vi "GC_GaN.vi"() -> ()   [LabVIEW 2011]
uses:
  DynaGlbs.vi
  ScrnGlbs.vi
  SysGlbs.vi
  TimeGlbs.vi
  SpecGlbs.vi
  RcpGlbs.vi
  RobotGlbs.vi
panel:
  out "PP Rout":string="Pump Purge Rout"
  out "shutter_indicator":string
  in  "32":bool
  in  "91":bool
  in  "92":bool
  in  "97":bool
  in  "101":bool
  in  "108":bool
  in  "123":bool
  out "val102 2":bool
  in  "Fout25":dbl min=0.0 max=5000.0 format="%.1f"
  in  "Fout29":dbl min=0.0 max=5000.0 format="%.1f"
  in  "Fout30":dbl min=0.0 max=5000.0 format="%.1f"
  in  "Fout26":dbl min=0.0 max=5000.0 format="%.1f"
  in  "Fout52":dbl min=0.0 max=5000.0 format="%.1f"
  in  "Fout53":dbl min=0.0 max=5000.0 format="%.1f"
  in  "Fout54":dbl min=0.0 max=5000.0 format="%.1f"
  in  "Fout38":dbl min=0.0 max=5000.0 format="%.1f"
  in  "Fout41":dbl min=0.0 max=5000.0 format="%.1f"
  in  "Fout49":dbl min=0.0 max=5000.0 format="%.1f"
  in  "Fout50":dbl min=0.0 max=5000.0 format="%.1f"
  in  "Fout51":dbl min=0.0 max=5000.0 format="%.1f"
  in  "Fout73":dbl min=0.0 max=5000.0 format="%.1f"
  in  "Fout87":dbl min=0.0 max=5000.0 format="%.1f"
  in  "Fout84":dbl min=0.0 max=5000.0 format="%.1f"
  in  "Fout83":dbl min=0.0 max=5000.0 format="%.1f"
  in  "Fout88":dbl min=0.0 max=5000.0 format="%.1f"
  in  "Fout74":dbl min=0.0 max=5000.0 format="%.1f"
  in  "Fout75":dbl min=0.0 max=5000.0 format="%.1f"
  in  "Fout76":dbl min=0.0 max=5000.0 format="%.1f"
  in  "Fout85":dbl min=0.0 max=5000.0 format="%.1f"
  in  "Fout55":dbl min=0.0 max=5000.0 format="%.1f"
  out "Fin84":dbl format="%.1f"
  out "Fin88":dbl format="%.1f"
  out "Fin83":dbl format="%.1f"
  out "Fin87":dbl format="%.1f"
  out "Fin86":dbl format="%.1f"
  out "Fin85":dbl format="%.1f"
  out "Fin92":dbl format="%.1f"
  out "Fin93":dbl format="%.1f"
  out "Fin94":dbl format="%.1f"
  out "Fin60":dbl format="%.3e"
  out "Fin61":dbl format="%.3e"
  out "Fin65":dbl format="%.1f"
  out "Fin73":dbl format="%.1f"
  out "Fin66":dbl format="%.1f"
  out "Fin67":dbl format="%.1f"
  out "Fin68":dbl format="%.1f"
  out "Fin69":dbl format="%.1f"
  out "Fin70":dbl format="%.1f"
  out "Fin74":dbl format="%.1f"
  out "Fin75":dbl format="%.1f"
  out "Fin76":dbl format="%.1f"
  out "Fin27":dbl format="%.1f"
  out "Fin29 2":dbl format="%.1f"
  out "Fin30 2":dbl format="%.1f"
  out "Fin38 2":dbl format="%.1f"
  out "Fin42 2":dbl format="%.1f"
  out "Fin52":dbl format="%.1f"
  out "Fin53":dbl format="%.1f"
  out "Fin54":dbl format="%.1f"
  out "Fin43":dbl format="%.1f"
  out "Fin41 2":dbl format="%.1f"
  out "Fin25 2":dbl format="%.1f"
  out "Fin26 2":dbl format="%.1f"
  out "Fin40":dbl format="%.1f"
  out "Fin49":dbl format="%.1f"
  out "Fin50":dbl format="%.1f"
  out "Fin51":dbl format="%.1f"
  out "Fin28":dbl format="%.1f"
  out "Fin55":dbl format="%.1f"
  in  "104":bool
  in  "ChgPW":bool
  in  "111":bool
  in  "110":bool
  in  "109":bool
  in  "112":bool
  in  "54":bool
  in  "Scrn Btns":T1
  out "bub8":string="TMAl #2"
  out "bub7":string="TMGa"
  out "bub6":string="TEGa"
  out "bub5":string="TMIn #2"
  out "bub4":string="TMIn #1"
  out "bub3":string="TMAl #1"
  out "bub2":string="Cp2Mg"
  out "bub1":string="DEZn"
  out "gas2":string="SiH4"
  in  "panel location and size":T2={"left"=0, "top"=78, "right"=887, "bottom"=700}
  in  "37":bool
  in  "38":bool
  in  "34":bool
  in  "36":bool
  in  "33":bool
  in  "35":bool
  in  "43":bool
  out "Vac lock":string="locked"
  out "LL lock":string="locked"
  out "GV lock":string="locked"
  in  "50":bool
  in  "49":bool
  out "LL Door":bool
  in  "44":bool
  in  "46":bool
  in  "40":bool
  in  "56":bool
  in  "42":bool
  in  "93":bool
  in  "39":bool
  in  "41":bool
  in  "47":bool
  in  "26":bool
  in  "53":bool
  in  "45":bool
  in  "55":bool
  in  "GV Down":bool=TRUE
  in  "GV Up":bool
  in  "30":bool
  in  "31":bool
  in  "94":bool
  in  "51":bool
  in  "103":bool
  in  "48":bool
  in  "28":bool
  in  "val102":bool
  in  "52":bool
  # "102"
  # "INNER"
  # "MIDDLE"
  # "OUTER"
  # "VOLTAGE"
  # "CURRENT"
  # "POWER"
  # "VIEW PORT\n   SHIELD"
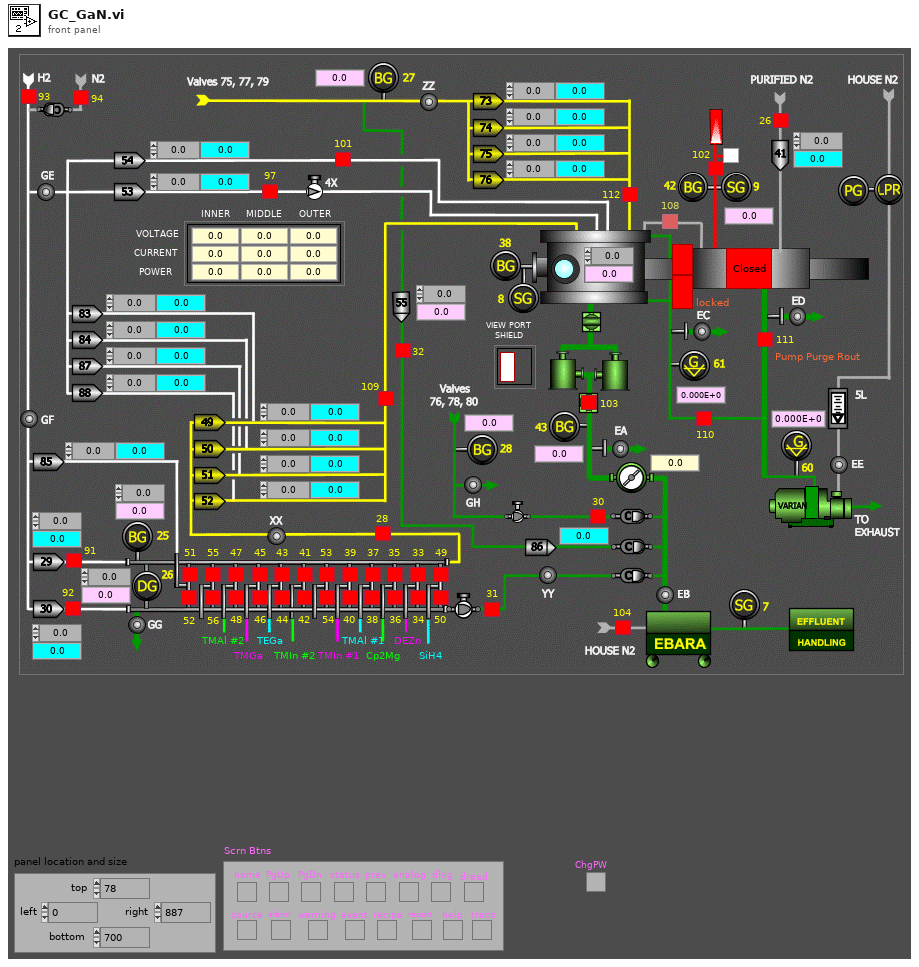
[diagram p1: front panel]
types:
  T1 = cluster{"home":bool, "PgUp":bool, "PgDn":bool, "status":bool, "prev":bool, "analog":bool, "dlog":bool, "dread":bool, "source":bool, "alarm":bool, "warning":bool, "event":bool, "recipe":bool, "report":bool, "help":bool, "trans":bool}
  T2 = cluster{"left":i16, "top":i16, "right":i16, "bottom":i16}
  T3 = enum16{"Load", "Read", "Open", "Close", "Invisible"}
  T4 = cluster{"Press":u8[], "PD_cell":cluster{"H2_cell":u8, "H2_line":u8, "horn":u8, "light":u8, "temp":u8, "PD_cell?":bool, "Temp Set":u16, "N2_in":u8, "N2_line":u8}, "RampDn":u8[], "GV/LL":cluster{"LL Door":u8, "GV Up":u8, "GV Low":u8, "GV _LIn":u8, "Fork":u8, "GV_UIn":u8, "GC Press":u8, "LL Press":u8, "MDA_LL":u8[], "Motor":u8, "EQ Valve":u8, "LL Active":u8}, "GC_Pump":cluster{"LL_Vac":u8, "GC_Vac":u8, "Bypass":u8, "Rough":u8, "Isolat":u8, "LL_MDA":u8[], "Vac_Press":u8, "TGV":u8}, "N2 Purge":cluster{"N2_LL":u8, "MFC":u8}, "RampRate":dbl[], "GC_Vac":cluster{"D_Vac-":u8[], "D_Vac+":u8[], "A_Vac":u8[], "D_Open+":u8[], "D_Open-":u8[], "A_Open":u8[]}, "Toxic":u8[], "Indicators":u8[], "LL Routine":cluster{"D Open":u8[], "D Close":u8[], "Timeout(ms)":u32}, "Temperature":u8[], "EBARA Pump":cluster{"EBARA_Din":cluster{"Main Status":u8, "Booster Status":u8, "Indicator":u8, "N2 Isolat":u8}, "EBARA_N2":u8[]}}
  T5 = cluster{"LL Door":u8, "GV Up":u8, "GV Low":u8, "GV _LIn":u8, "Fork":u8, "GV_UIn":u8, "GC Press":u8, "LL Press":u8, "MDA_LL":u8[], "Motor":u8, "EQ Valve":u8, "LL Active":u8}
  T6 = cluster{"[0]":dbl, "[1]":dbl, "[2]":dbl, "[3]":dbl, "[4]":dbl, "[5]":dbl}
  T7 = cluster{"[0]":dbl, "[1]":dbl, "[2]":dbl, "[3]":dbl, "[4]":dbl, "[5]":dbl, "[6]":dbl}
  T8 = cluster{"[0]":dbl, "[1]":dbl, "[2]":dbl, "[3]":dbl, "[4]":dbl, "[5]":dbl, "[6]":dbl, "[7]":dbl, "[8]":dbl, "[9]":dbl, "[10]":dbl}
  T9 = cluster{"[0]":dbl, "[1]":dbl, "[2]":dbl, "[3]":dbl}
  T10 = enum16{"Init", "Check", "TGA Status", "TGA Scrn", "Read"}
  T11 = cluster{"[0]":bool, "[1]":bool, "[2]":bool, "[3]":bool, "[4]":bool, "[5]":bool, "[6]":bool, "[7]":bool, "[8]":bool, "[9]":bool, "[10]":bool, "[11]":bool, "[12]":bool, "[13]":bool, "[14]":bool, "[15]":bool, "[16]":bool, "[17]":bool, "[18]":bool, "[19]":bool, "[20]":bool, "[21]":bool, "[22]":bool, "[23]":bool, "[24]":bool, "[25]":bool, "[26]":bool, "[27]":bool, "[28]":bool, "[29]":bool, "[30]":bool, "[31]":bool, "[32]":bool, "[33]":bool, "[34]":bool, "[35]":bool}
  T12 = cluster{"[0]":bool, "[1]":bool, "[2]":bool, "[3]":bool}
  T13 = cluster{"[0]":bool, "[1]":bool, "[2]":bool, "[3]":bool, "[4]":bool}
  T14 = cluster{"[0]":bool, "[1]":bool, "[2]":bool, "[3]":bool, "[4]":bool, "[5]":bool}
  T15 = cluster{"[0]":bool, "[1]":bool, "[2]":bool, "[3]":bool, "[4]":bool, "[5]":bool, "[6]":bool}
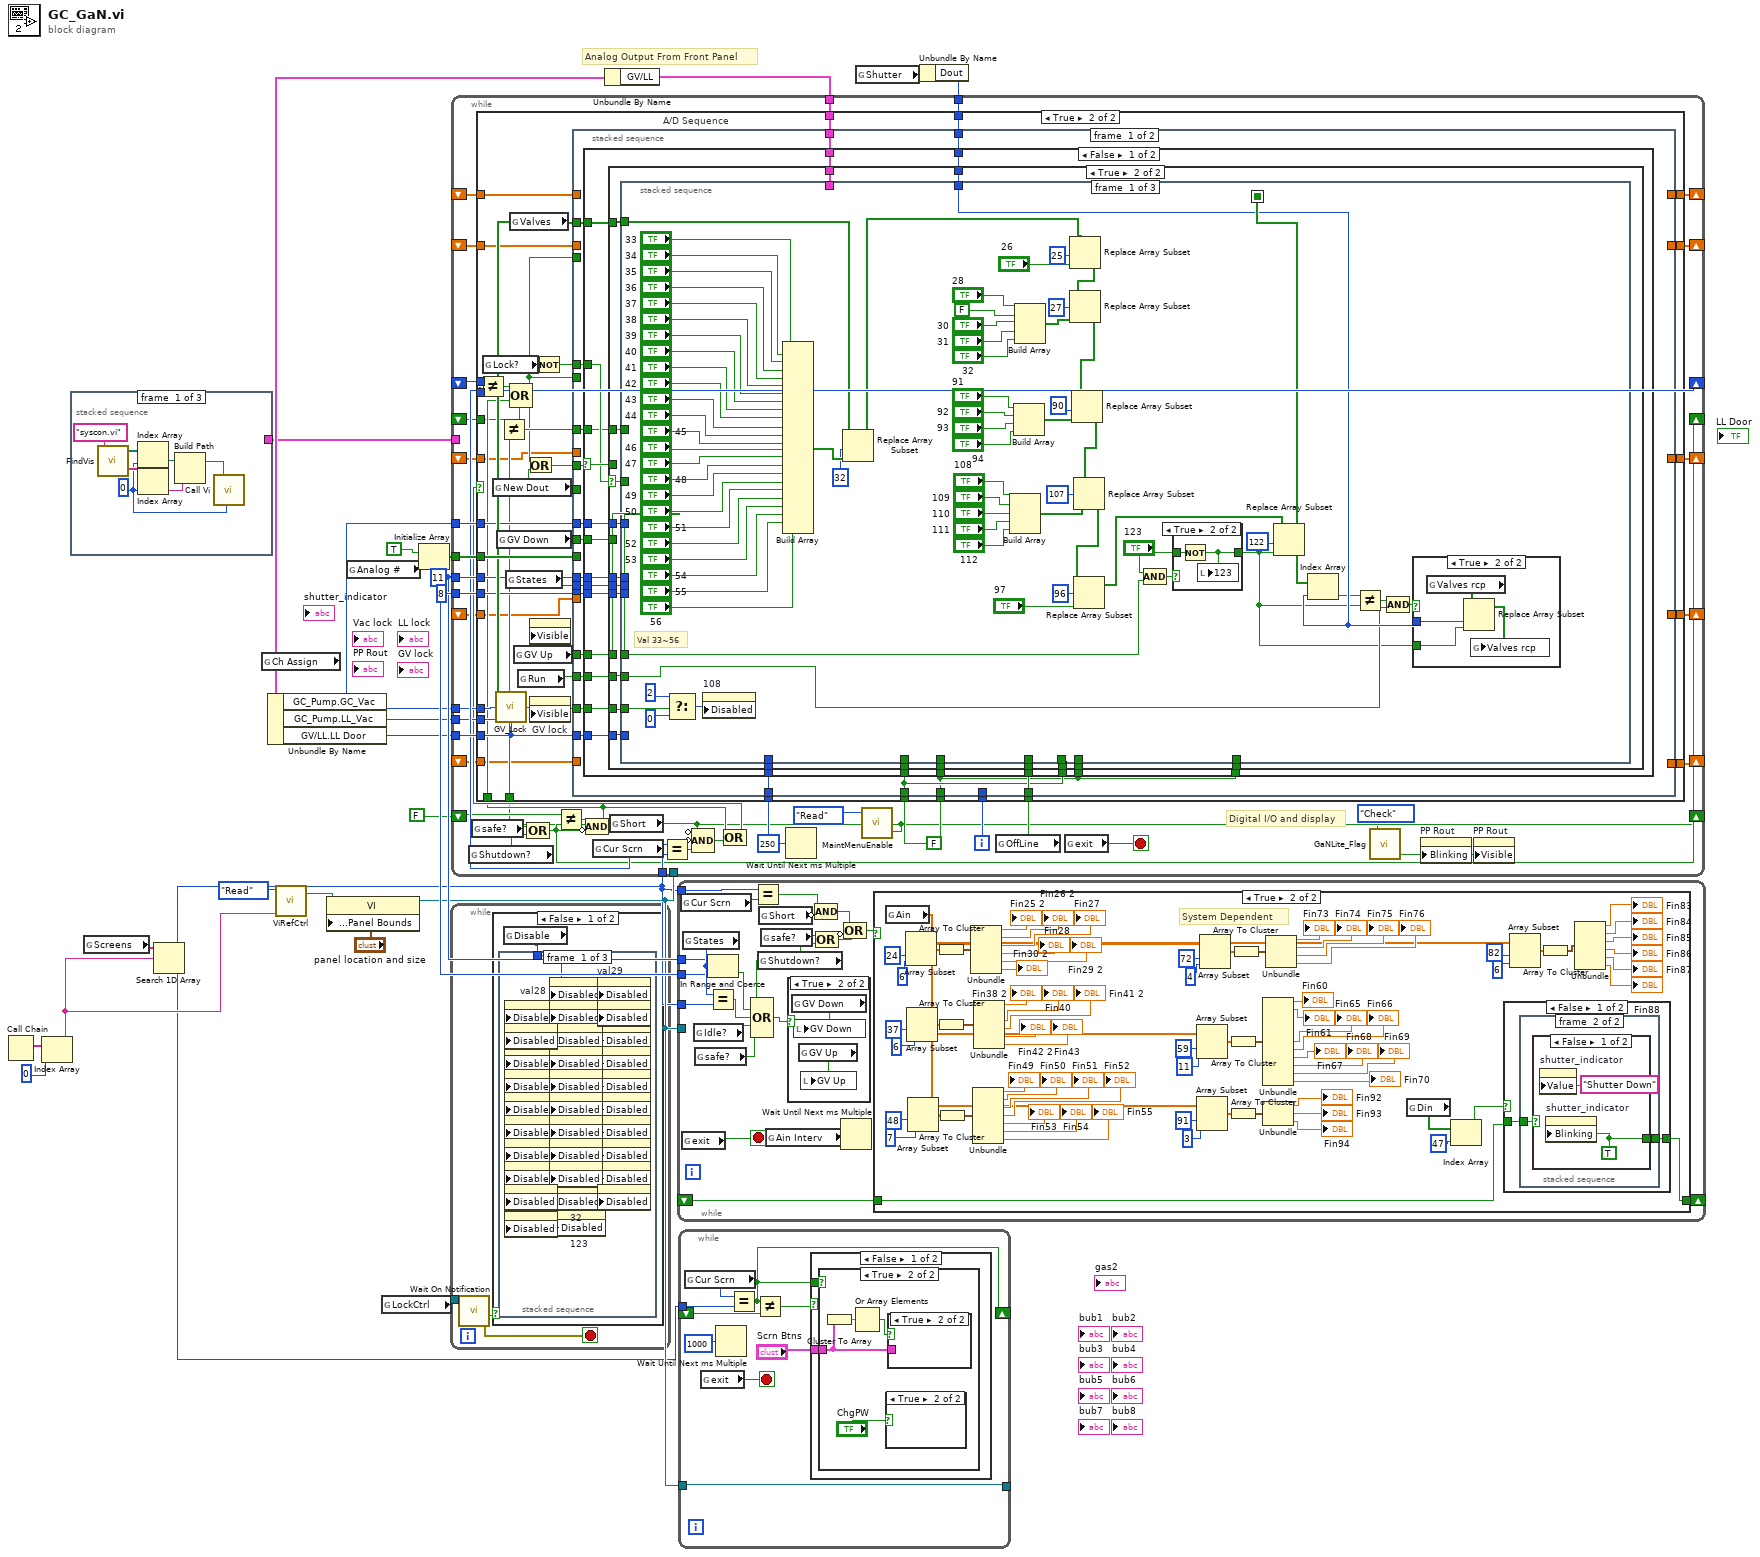
[diagram p0: block diagram]
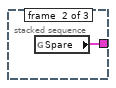
[diagram p2: hidden frame]
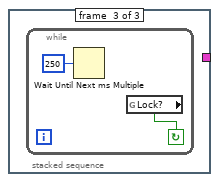
[diagram p3: hidden frame]
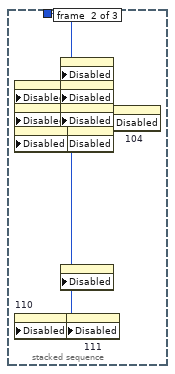
[diagram p4: hidden frame]
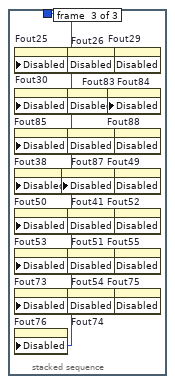
[diagram p5: hidden frame]
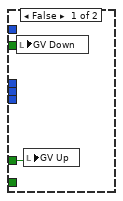
[diagram p12: hidden frame]
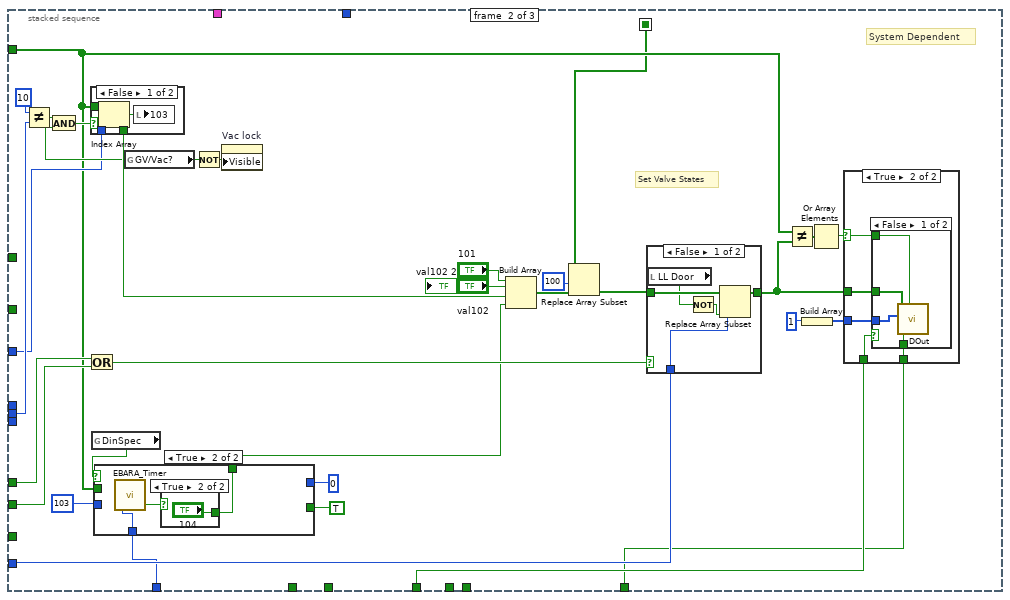
[diagram p15: hidden frame]
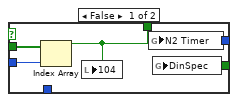
[diagram p16: hidden frame]
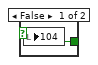
[diagram p17: hidden frame]
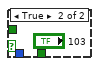
[diagram p18: hidden frame]
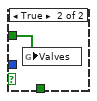
[diagram p20: hidden frame]
diagram:
  w20 = 11
  w21 = 8
  # "Analog Output From Front Panel"
  n1 = Call Chain() -> (call chain=w6:string[])
  n2 = Index Array(array=w6, index=0) -> (element=w4:string)
  n3 = stacked-sequence {
    tunnel: [_ w32 _] -> w10
    frame #0 {
      w25 = 0
      n4 = call "FindVis.vi"("Caller"="syscon.vi") -> ("Subllbs"=w30:path[], "SubVis"=w29:string[])
      n5 = Index Array(array=w30, index=w25) -> (element=w28:path)
      n6 = Index Array(array=w29, index=w25) -> (element=w27:string)
      n7 = Build Path(base path=w28, name or relative path=w27) -> (appended path=w26:path)
      n8 = call "Call Vi.vi"("call mode (open,call,close:1)"=w25, "VI path"=w26) -> ()  [unwired: 8 in, 2 out]
    }
    frame #1 {
      n9 = global read "SpecGlbs.vi" "Spare"() -> (w32:cluster{"SpareD":bool[], "SpareA":bool[]})
    }
    frame #2 {
      n10 = while {
        stop <- w34 continue-if-true
        n11 = Wait Until Next ms Multiple(millisecond multiple=u32 250) -> ()  [unwired: 1 out]
        n12 = global read "ScrnGlbs.vi" "Lock?"() -> (w34:bool)
      }
    }
  }
  n13 = global read "ScrnGlbs.vi" "Screens"() -> (w7:string[])
  n14 = Search 1D Array(1D array=w7, element=w4) -> (index of element=w3:i32)  [unwired: 1 in]
  n15 = global read "SysGlbs.vi" "Ch Assign"() -> (w13:T4)
  n16 = Unbundle By Name(w13) -> ("GC_Pump.GC_Vac"=w18:u8, "GC_Pump.LL_Vac"=w17:u8, "GV/LL.LL Door"=w16:u8)
  n17 = call "ViRefCtrl.vi"("Action"=T3."Read", "Vi Name"=w4) -> ("Vi Ref"=w14:refnum<vi>)  [unwired: 3 in, 1 out]
  n18 = property class="VI"(reference=w14, "Front Panel Window:Panel Bounds"="panel location and size") -> (reference out=w12:refnum<vi>)  [unwired: 1 in, 1 out]
  n19 = global read "SysGlbs.vi" "Analog #"() -> (w22:u32)
  n20 = global read "ScrnGlbs.vi" "LockCtrl"() -> (w11:refnum<k1>)
  n21 = Initialize Array(TRUE, w22) -> (w23:bool[])
  n22 = while {
    tunnel: w11 -> [w37]
    stop <- w35 stop-if-true
    n23 = call <vilib>:"Wait On Notification.vi"("notifier"=w37) -> ("error out"=w35:errorcluster, "timed out"=w36:bool)  [unwired: 3 in, 2 out]
    n24 = case shown="False" w36 {
      frame False {
        n25 = global read "ScrnGlbs.vi" "Disable"() -> (w38:u8)
        n26 = stacked-sequence {
          tunnel: w38 -> [w39 w40 w41]
          frame #0 {
            n27 = property on="val30" class="Bool (strict)"("Disabled"=w39) -> ()  [unwired: 2 in, 2 out]
            n28 = property on="34" class="Bool (strict)"("Disabled"=w39) -> ()  [unwired: 2 in, 2 out]
            n29 = property on="val36" class="Bool (strict)"("Disabled"=w39) -> ()  [unwired: 2 in, 2 out]
            n30 = property on="val39" class="Bool (strict)"("Disabled"=w39) -> ()  [unwired: 2 in, 2 out]
            n31 = property on="val42" class="Bool (strict)"("Disabled"=w39) -> ()  [unwired: 2 in, 2 out]
            n32 = property on="val45" class="Bool (strict)"("Disabled"=w39) -> ()  [unwired: 2 in, 2 out]
            n33 = property on="val48" class="Bool (strict)"("Disabled"=w39) -> ()  [unwired: 2 in, 2 out]
            n34 = property on="val51" class="Bool (strict)"("Disabled"=w39) -> ()  [unwired: 2 in, 2 out]
            n35 = property on="54" class="Bool (strict)"("Disabled"=w39) -> ()  [unwired: 2 in, 2 out]
            n36 = property on="112" class="Bool (strict)"("Disabled"=w39) -> ()  [unwired: 2 in, 2 out]
            n37 = property on="val28" class="Bool (strict)"("Disabled"=w39) -> ()  [unwired: 2 in, 2 out]
            n38 = property on="val31" class="Bool (strict)"("Disabled"=w39) -> ()  [unwired: 2 in, 2 out]
            n39 = property on="val37" class="Bool (strict)"("Disabled"=w39) -> ()  [unwired: 2 in, 2 out]
            n40 = property on="val40" class="Bool (strict)"("Disabled"=w39) -> ()  [unwired: 2 in, 2 out]
            n41 = property on="val43" class="Bool (strict)"("Disabled"=w39) -> ()  [unwired: 2 in, 2 out]
            n42 = property on="val46" class="Bool (strict)"("Disabled"=w39) -> ()  [unwired: 2 in, 2 out]
            n43 = property on="val49" class="Bool (strict)"("Disabled"=w39) -> ()  [unwired: 2 in, 2 out]
            n44 = property on="val52" class="Bool (strict)"("Disabled"=w39) -> ()  [unwired: 2 in, 2 out]
            n45 = property on="val55" class="Bool (strict)"("Disabled"=w39) -> ()  [unwired: 2 in, 2 out]
            n46 = property on="32" class="Bool (strict)"("Disabled"=w39) -> ()  [unwired: 2 in, 2 out]
            n47 = property on="123" class="Bool (strict)"("Disabled"=w39) -> ()  [unwired: 2 in, 2 out]
            n48 = property on="val29" class="Bool (strict)"("Disabled"=w39) -> ()  [unwired: 2 in, 2 out]
            n49 = property on="33" class="Bool (strict)"("Disabled"=w39) -> ()  [unwired: 2 in, 2 out]
            n50 = property on="val35" class="Bool (strict)"("Disabled"=w39) -> ()  [unwired: 2 in, 2 out]
            n51 = property on="val38" class="Bool (strict)"("Disabled"=w39) -> ()  [unwired: 2 in, 2 out]
            n52 = property on="val41" class="Bool (strict)"("Disabled"=w39) -> ()  [unwired: 2 in, 2 out]
            n53 = property on="val44" class="Bool (strict)"("Disabled"=w39) -> ()  [unwired: 2 in, 2 out]
            n54 = property on="val47" class="Bool (strict)"("Disabled"=w39) -> ()  [unwired: 2 in, 2 out]
            n55 = property on="val50" class="Bool (strict)"("Disabled"=w39) -> ()  [unwired: 2 in, 2 out]
            n56 = property on="val53" class="Bool (strict)"("Disabled"=w39) -> ()  [unwired: 2 in, 2 out]
            n57 = property on="val56" class="Bool (strict)"("Disabled"=w39) -> ()  [unwired: 2 in, 2 out]
          }
          frame #1 {
            n58 = property on="val93" class="Bool (strict)"("Disabled"=w40) -> ()  [unwired: 2 in, 2 out]
            n59 = property on="GV Up" class="Bool (strict)"("Disabled"=w40) -> ()  [unwired: 2 in, 2 out]
            n60 = property on="val102" class="Bool (strict)"("Disabled"=w40) -> ()  [unwired: 2 in, 2 out]
            n61 = property on="110" class="Bool (strict)"("Disabled"=w40) -> ()  [unwired: 2 in, 2 out]
            n62 = property on="val94" class="Bool (strict)"("Disabled"=w40) -> ()  [unwired: 2 in, 2 out]
            n63 = property on="LL Door" class="Bool (strict)"("Disabled"=w40) -> ()  [unwired: 2 in, 2 out]
            n64 = property on="GV Down" class="Bool (strict)"("Disabled"=w40) -> ()  [unwired: 2 in, 2 out]
            n65 = property on="val103" class="Bool (strict)"("Disabled"=w40) -> ()  [unwired: 2 in, 2 out]
            n66 = property on="109" class="Bool (strict)"("Disabled"=w40) -> ()  [unwired: 2 in, 2 out]
            n67 = property on="111" class="Bool (strict)"("Disabled"=w40) -> ()  [unwired: 2 in, 2 out]
            n68 = property on="104" class="Bool (strict)"("Disabled"=w40) -> ()  [unwired: 2 in, 2 out]
          }
          frame #2 {
            n69 = property on="Fout25" class="DigNum (strict)"("Disabled"=w41) -> ()  [unwired: 2 in, 2 out]
            n70 = property on="Fout30" class="DigNum (strict)"("Disabled"=w41) -> ()  [unwired: 2 in, 2 out]
            n71 = property on="Fout85" class="DigNum (strict)"("Disabled"=w41) -> ()  [unwired: 2 in, 2 out]
            n72 = property on="Fout38" class="DigNum (strict)"("Disabled"=w41) -> ()  [unwired: 2 in, 2 out]
            n73 = property on="Fout50" class="DigNum (strict)"("Disabled"=w41) -> ()  [unwired: 2 in, 2 out]
            n74 = property on="Fout53" class="DigNum (strict)"("Disabled"=w41) -> ()  [unwired: 2 in, 2 out]
            n75 = property on="Fout73" class="DigNum (strict)"("Disabled"=w41) -> ()  [unwired: 2 in, 2 out]
            n76 = property on="Fout76" class="DigNum (strict)"("Disabled"=w41) -> ()  [unwired: 2 in, 2 out]
            n77 = property on="Fout26" class="DigNum (strict)"("Disabled"=w41) -> ()  [unwired: 2 in, 2 out]
            n78 = property on="Fout83" class="DigNum (strict)"("Disabled"=w41) -> ()  [unwired: 2 in, 2 out]
            n79 = property on="Fout87" class="DigNum (strict)"("Disabled"=w41) -> ()  [unwired: 2 in, 2 out]
            n80 = property on="Fout41" class="DigNum (strict)"("Disabled"=w41) -> ()  [unwired: 2 in, 2 out]
            n81 = property on="Fout51" class="DigNum (strict)"("Disabled"=w41) -> ()  [unwired: 2 in, 2 out]
            n82 = property on="Fout54" class="DigNum (strict)"("Disabled"=w41) -> ()  [unwired: 2 in, 2 out]
            n83 = property on="Fout74" class="DigNum (strict)"("Disabled"=w41) -> ()  [unwired: 2 in, 2 out]
            n84 = property on="Fout29" class="DigNum (strict)"("Disabled"=w41) -> ()  [unwired: 2 in, 2 out]
            n85 = property on="Fout84" class="DigNum (strict)"("Disabled"=w41) -> ()  [unwired: 2 in, 2 out]
            n86 = property on="Fout88" class="DigNum (strict)"("Disabled"=w41) -> ()  [unwired: 2 in, 2 out]
            n87 = property on="Fout49" class="DigNum (strict)"("Disabled"=w41) -> ()  [unwired: 2 in, 2 out]
            n88 = property on="Fout52" class="DigNum (strict)"("Disabled"=w41) -> ()  [unwired: 2 in, 2 out]
            n89 = property on="Fout55" class="DigNum (strict)"("Disabled"=w41) -> ()  [unwired: 2 in, 2 out]
            n90 = property on="Fout75" class="DigNum (strict)"("Disabled"=w41) -> ()  [unwired: 2 in, 2 out]
          }
        }
      }
      frame True {
      }
    }
  }
  n91 = Unbundle By Name(w13) -> ("GV/LL"=w19:T5)
  n92 = while {
    tunnel: w12 -> [_]
    tunnel: w3 -> [w61]
    tunnel: w21 -> [w59]
    tunnel: w3 -> [w58]
    tunnel: w20 -> [w57]
    shift-right: [w42] -> _
    shift-left: _ -> [w43]
    stop <- w44 stop-if-true
    n93 = global read "ScrnGlbs.vi" "Cur Scrn"() -> (w62:i32)
    n94 = global read "ScrnGlbs.vi" "exit"() -> (w44:bool)
    n95 = global read "DynaGlbs.vi" "States"() -> (w60:u8)
    n96 = global read "ScrnGlbs.vi" "Idle?"() -> (w53:bool)
    n97 = global read "ScrnGlbs.vi" "safe?"() -> (w52:bool)
    n98 = In Range and Coerce(upper limit=w57, x=w60, lower limit=w59) -> (In Range?=w56:bool)  [unwired: 1 out]
    n99 = Equal?(x=w60, y=w58) -> (x = y?=w55:bool)
    n100 = Equal?(x=w61, y=w62) -> (x = y?=w51:bool)
    n101 = global read "ScrnGlbs.vi" "Shutdown?"() -> (w46:bool)
    n102 = Compound Arithmetic op=OR(w46, w56, w55, w53, w52) -> (w54:bool)
    n103 = global read "TimeGlbs.vi" "Short"() -> (w50:bool)
    n104 = global read "ScrnGlbs.vi" "safe?"() -> (w47:bool)
    n105 = global read "TimeGlbs.vi" "Ain Interv"() -> (w63:u32)
    n106 = case shown="True" w54 {
      frame False {
      }
      frame True {
        n107 = global read "ScrnGlbs.vi" "GV Down"() -> (w65:bool)
        n108 = local write "GV Down"(w65) -> ()
        n109 = global read "ScrnGlbs.vi" "GV Up"() -> (w64:bool)
        n110 = local write "GV Up"(w64) -> ()
      }
    }
    n111 = Compound Arithmetic op=AND(w51, invert w50) -> (w49:bool)
    n112 = Compound Arithmetic op=OR(w47, w46) -> (w45:bool)
    n113 = Wait Until Next ms Multiple(millisecond multiple=w63) -> ()  [unwired: 1 out]
    n114 = Compound Arithmetic op=OR(w49, invert w45) -> (w48:bool)
    n115 = case shown="True" w48 {
      tunnel: w43 -> [w66 w68]
      tunnel: [w66 w67] -> w42
      frame False {
      }
      frame True {
        # "System Dependent"
        n116 = global read "DynaGlbs.vi" "Ain"() -> (w72:dbl[])
        n117 = Array Subset(array=w72, index=24, length=6) -> (w134:dbl[])
        n118 = Array Subset(array=w72, index=37, length=6) -> (w133:dbl[])
        n119 = Array Subset(array=w72, index=48, length=7) -> (w131:dbl[])
        n120 = Array To Cluster(array=w134) -> (cluster=w139:T6)
        n121 = Array To Cluster(array=w133) -> (cluster=w137:T6)
        n122 = Array To Cluster(array=w131) -> (cluster=w138:T7)
        n123 = Unbundle(w139) -> ("[0]"=→"Fin25 2":dbl, "[1]"=→"Fin26 2":dbl, "[2]"=→"Fin27":dbl, "[3]"=→"Fin28":dbl, "[4]"=→"Fin29 2":dbl, "[5]"=→"Fin30 2":dbl)
        n124 = Unbundle(w138) -> ("[0]"=→"Fin49":dbl, "[1]"=→"Fin50":dbl, "[2]"=→"Fin51":dbl, "[3]"=→"Fin52":dbl, "[4]"=→"Fin53":dbl, "[5]"=→"Fin54":dbl, "[6]"=→"Fin55":dbl)
        n125 = Unbundle(w137) -> ("[0]"=→"Fin38 2":dbl, "[2]"=→"Fin40":dbl, "[3]"=→"Fin41 2":dbl, "[4]"=→"Fin42 2":dbl, "[5]"=→"Fin43":dbl)  [unwired: 1 out]
        n126 = Array Subset(array=w72, index=59 ("Array Index"), length=11 ("Array Length")) -> (w120:dbl[])
        n127 = Array Subset(array=w72, index=91 ("Array Index"), length=3 ("Array Length")) -> (w128:dbl[])
        n128 = Array Subset(array=w72, index=72 ("Array Index"), length=4 ("Array Length")) -> (w115:dbl[])
        n129 = Array To Cluster(array=w120) -> (cluster=w121:T8)
        n130 = Array To Cluster(array=w128) -> (cluster=w129:cluster{"[0]":dbl, "[1]":dbl, "[2]":dbl})
        n131 = Array To Cluster(array=w115) -> (cluster=w114:T9)
        n132 = Unbundle(w121) -> ("[0]"=→"Fin60":dbl, "[1]"=→"Fin61":dbl, "[5]"=→"Fin65":dbl, "[6]"=→"Fin66":dbl, "[7]"=→"Fin67":dbl, "[8]"=→"Fin68":dbl, "[9]"=→"Fin69":dbl, "[10]"=→"Fin70":dbl)  [unwired: 3 out]
        n133 = Unbundle(w129) -> ("[0]"=→"Fin92":dbl, "[1]"=→"Fin93":dbl, "[2]"=→"Fin94":dbl)
        n134 = Unbundle(w114) -> ("[0]"=→"Fin73":dbl, "[1]"=→"Fin74":dbl, "[2]"=→"Fin75":dbl, "[3]"=→"Fin76":dbl)
        n135 = global read "DynaGlbs.vi" "Din"() -> (w71:bool[])
        n136 = Index Array(array=w71, index=47 ("Index")) -> (element=w69:bool)
        n137 = case shown="False" w69 {
          tunnel: [w141 w150] -> w67
          tunnel: w68 -> [w140 w150]
          frame False {
            n138 = stacked-sequence {
              tunnel: [_ w144] -> w141
              tunnel: w140 -> [_ w143]
              frame #0 {
                n139 = property on="shutter_indicator" class="Str"("Visible"=TRUE) -> ()  [unwired: 2 in, 2 out]
              }
              frame #1 {
                n140 = case shown="False" w143 {
                  selector: w143 -> [_ w148]
                  tunnel: [w145 w148] -> w144
                  frame False {
                    w145 = TRUE
                    n141 = property on="shutter_indicator" class="Str"("Value"="Shutter Down") -> ()  [unwired: 2 in, 2 out]
                    n142 = property on="shutter_indicator" class="Str"("Blinking"=w145) -> ()  [unwired: 2 in, 2 out]
                  }
                  frame True {
                    n143 = property on="shutter_indicator" class="Str"("Value"="Shutter Down") -> ()  [unwired: 2 in, 2 out]
                  }
                }
              }
            }
          }
          frame True {
            n144 = property on="shutter_indicator" class="Str"("Visible"=FALSE) -> ()  [unwired: 2 in, 2 out]
          }
        }
        n145 = Array Subset(array=w72, index=82 ("Array Index"), length=6 ("Array Length")) -> (w122:dbl[])
        n146 = Array To Cluster(array=w122) -> (cluster=w123:T6)
        n147 = Unbundle(w123) -> ("[0]"=→"Fin83":dbl, "[1]"=→"Fin84":dbl, "[2]"=→"Fin85":dbl, "[3]"=→"Fin86":dbl, "[4]"=→"Fin87":dbl, "[5]"=→"Fin88":dbl)
      }
    }
  }
  n148 = while {
    shift-right: [w157] -> _
    shift-left: _ -> [w158]
    tunnel: w12 -> [w156]
    tunnel: [w156] -> _
    tunnel: w3 -> [w152]
    stop <- w151 stop-if-true
    n149 = global read "ScrnGlbs.vi" "Cur Scrn"() -> (w155:i32)
    n150 = global read "ScrnGlbs.vi" "exit"() -> (w151:bool)
    n151 = Wait Until Next ms Multiple(millisecond multiple=u32 1000) -> ()  [unwired: 1 out]
    n152 = Equal?(x=w155, y=w152) -> (x = y?=w157:bool)
    n153 = Not Equal?(x=w157, y=w158) -> (x != y?=w154:bool)
    n154 = case shown="False" w154 {
      tunnel: "Scrn Btns" -> [w160 _]
      tunnel: w157 -> [w161 _]
      frame False {
        n155 = case shown="True" w161 {
          tunnel: w160 -> [_ w163]
          frame False {
          }
          frame True {
            n156 = Cluster To Array(cluster=w163) -> (array=w164:bool[])
            n157 = Or Array Elements(Boolean array=w164) -> (logical OR=w165:bool)
            n158 = case shown="True" "ChgPW" {
              frame False {
              }
              frame True {
              }
            }
            n159 = case shown="True" w165 {
              tunnel: w163 -> [_ _]
              frame False {
              }
              frame True {
              }
            }
          }
        }
      }
      frame True {
      }
    }
  }
  n160 = global read "SysGlbs.vi" "Shutter"() -> (w2:cluster{"Din":i32, "Dout":i32})
  n161 = Unbundle By Name(w2) -> ("Dout"=w1:i32)
  n162 = while {
    tunnel: w23 -> [w206]
    tunnel: w16 -> [w205]
    tunnel: w12 -> [_]
    tunnel: w3 -> [w204]
    tunnel: w21 -> [w201]
    tunnel: w20 -> [w200]
    tunnel: w18 -> [w199]
    shift-right: [w197] -> _
    shift-left: _ -> [w198]
    tunnel: w19 -> [w196]
    tunnel: w18 -> [w195]
    tunnel: w17 -> [w194]
    tunnel: w10 -> [_]
    shift-right: [w185] -> _
    shift-left: FALSE -> [w186]
    shift-right: [w181] -> _
    shift-left: _ -> [w182]
    tunnel: w1 -> [w179]
    shift-right: [w171] -> _
    shift-left: _ -> [w175]
    shift-right: [w176] -> _
    shift-left: _ -> [w177]
    shift-right: [w170] -> _
    shift-left: _ -> [w174]
    shift-right: [w169] -> _
    shift-left: _ -> [w173]
    shift-right: [w168] -> _
    shift-left: _ -> [w172]
    i -> [w193]
    stop <- w180 stop-if-true
    w202 = FALSE
    w207 = u32 250
    # "Digital I/O and display"
    n163 = global read "ScrnGlbs.vi" "Shutdown?"() -> (w183:bool)
    n164 = global read "ScrnGlbs.vi" "safe?"() -> (w184:bool)
    n165 = Compound Arithmetic op=OR(w184, w183) -> (w185:bool)
    n166 = Not Equal?(x=w186, y=w185) -> (x != y?=w188:bool)
    n167 = Compound Arithmetic op=AND(w188, invert w185) -> (w187:bool)
    n168 = global read "ScrnGlbs.vi" "Cur Scrn"() -> (w197:i32)
    n169 = global read "TimeGlbs.vi" "Short"() -> (w192:bool)
    n170 = Equal?(x=w197, y=w204) -> (x = y?=w191:bool)
    n171 = Wait Until Next ms Multiple(millisecond multiple=w207) -> ()  [unwired: 1 out]
    n172 = call "MaintMenuEnable.vi"("Action"=T10."Read") -> ("Maint Active"=w181:bool)  [unwired: 3 in, 1 out]
    n173 = Compound Arithmetic op=AND(invert w181, invert w192, w191) -> (w190:bool)
    n174 = Compound Arithmetic op=OR(w187, w190) -> (w189:bool)
    n175 = global read "ScrnGlbs.vi" "OffLine"() -> (w203:bool)
    n176 = case shown="True" w189 {
      tunnel: w206 -> [_ w253]
      tunnel: w205 -> [_ w234]
      tunnel: w202 -> [_ w252]
      tunnel: w203 -> [_ w250]
      tunnel: w202 -> [_ w248]
      tunnel: w194 -> [_ w245]
      tunnel: w201 -> [_ w247]
      tunnel: w200 -> [_ w246]
      tunnel: w199 -> [_ w242]
      tunnel: w198 -> [_ w239]
      tunnel: w197 -> [_ w238]
      tunnel: w196 -> [_ w235]
      tunnel: w195 -> [_ w233]
      tunnel: w193 -> [_ w232]
      tunnel: w207 -> [_ w231]
      tunnel: w187 -> [_ w230]
      tunnel: w182 -> [_ w228]
      tunnel: w181 -> [_ w226]
      tunnel: w179 -> [_ w223]
      tunnel: w177 -> [w212 w222]
      tunnel: [w212 w221] -> w176
      tunnel: w175 -> [w211 w220]
      tunnel: w174 -> [w210 w219]
      tunnel: w173 -> [w209 w218]
      tunnel: w172 -> [w208 w217]
      tunnel: [w211 w216] -> w171
      tunnel: [w210 w215] -> w170
      tunnel: [w209 w214] -> w169
      tunnel: [w208 w213] -> w168
      frame False {
      }
      frame True {
        n177 = Not Equal?(x=w239, y=w238) -> (x != y?=w229:bool)
        n178 = global read "ScrnGlbs.vi" "Lock?"() -> (w241:bool)
        n179 = global read "DynaGlbs.vi" "New Dout"() -> (w237:bool)
        n180 = global read "ScrnGlbs.vi" "GV Down"() -> (w224:bool)
        n181 = Not Equal?(x=w228, y=w226) -> (x != y?=w227:bool)
        n182 = global read "DynaGlbs.vi" "States"() -> (w249:u8)
        n183 = global read "DynaGlbs.vi" "Valves"() -> (w251:bool[])
        n184 = call "GV_Lock.vi"("LL Door"=w234, "LL_Vac"=w245, "GC_Vac"=w233, "Valves"=w251) -> ("lock?"=w244:bool)
        n185 = Compound Arithmetic op=OR(w229, w230, w227) -> (w225:bool)
        n186 = global read "ScrnGlbs.vi" "GV Up"() -> (w243:bool)
        n187 = global read "ScrnGlbs.vi" "Run"() -> (w254:bool)
        n188 = Or(x=w225, y=w237) -> (x .or. y?=w236:bool)
        n189 = property on="LL lock" class="Str"("Visible"=w243) -> ()  [unwired: 2 in, 2 out]
        n190 = property on="GV lock" class="Str"("Visible"=w244) -> ()  [unwired: 2 in, 2 out]
        n191 = Not(x=w241) -> (.not. x?=w240:bool)
        n192 = stacked-sequence "A/D Sequence" {
          tunnel: w254 -> [w273 w625]
          tunnel: w252 -> [w258 w623]
          tunnel: w253 -> [_ w626]
          tunnel: w234 -> [w272 _]
          tunnel: w237 -> [_ _]
          tunnel: w251 -> [w271 _]
          tunnel: w250 -> [w270 w622]
          tunnel: w249 -> [w269 _]
          tunnel: w248 -> [w268 _]
          tunnel: w247 -> [w266 _]
          tunnel: w246 -> [w265 _]
          tunnel: w244 -> [w264 _]
          tunnel: w243 -> [w263 _]
          tunnel: w242 -> [w262 _]
          tunnel: w240 -> [w267 w621]
          tunnel: w236 -> [w261 _]
          tunnel: w225 -> [_ w617]
          tunnel: w235 -> [w260 _]
          tunnel: w232 -> [_ w620]
          tunnel: w231 -> [w259 _]
          tunnel: w225 -> [_ w614]
          tunnel: w224 -> [w257 _]
          tunnel: w227 -> [w256 _]
          tunnel: w223 -> [w255 _]
          tunnel: w222 -> [_ w610]
          tunnel: [_ w609] -> w221
          tunnel: w220 -> [_ w608]
          tunnel: w219 -> [_ w607]
          tunnel: w218 -> [_ w606]
          tunnel: w217 -> [_ w605]
          tunnel: [_ w604] -> w216
          tunnel: [_ w603] -> w215
          tunnel: [_ w602] -> w214
          tunnel: [_ w601] -> w213
          frame #0 {
            n193 = case shown="False" w261 {
              selector: w261 -> [w294 _]
              tunnel: w273 -> [w293 _]
              tunnel: w272 -> [w290 w597]
              tunnel: w258 -> [w292 w598]
              tunnel: w270 -> [w291 _]
              tunnel: w271 -> [w295 w534]
              tunnel: w269 -> [w278 _]
              tunnel: w258 -> [w289 _]
              tunnel: w268 -> [w288 _]
              tunnel: w267 -> [w280 _]
              tunnel: w266 -> [w277 _]
              tunnel: w265 -> [w279 _]
              tunnel: w264 -> [w287 _]
              tunnel: w263 -> [w286 _]
              tunnel: w268 -> [w285 _]
              tunnel: w262 -> [w284 _]
              tunnel: w260 -> [w283 _]
              tunnel: w259 -> [w282 _]
              tunnel: w258 -> [w281 _]
              tunnel: w257 -> [w276 _]
              tunnel: w256 -> [w275 _]
              tunnel: w255 -> [w274 _]
              frame False {
                n194 = case shown="True" w280 {
                  selector: w280 -> [_ w309]
                  tunnel: w295 -> [_ w317]
                  tunnel: w294 -> [_ _]
                  tunnel: w293 -> [_ w316]
                  tunnel: w290 -> [_ w315]
                  tunnel: w292 -> [_ w314]
                  tunnel: w291 -> [_ w313]
                  tunnel: w289 -> [_ w312]
                  tunnel: w288 -> [_ w311]
                  tunnel: w287 -> [_ w310]
                  tunnel: w286 -> [w297 w308]
                  tunnel: w285 -> [_ w307]
                  tunnel: w284 -> [_ w306]
                  tunnel: w283 -> [_ w305]
                  tunnel: w282 -> [_ w304]
                  tunnel: w281 -> [_ w303]
                  tunnel: w279 -> [_ w302]
                  tunnel: w278 -> [_ w301]
                  tunnel: w277 -> [_ w300]
                  tunnel: w276 -> [w296 _]
                  tunnel: w275 -> [_ w299]
                  tunnel: w274 -> [_ w298]
                  frame False {
                    n195 = local write "GV Down"(w296) -> ()
                    n196 = local write "GV Up"(w297) -> ()
                  }
                  frame True {
                    n197 = stacked-sequence {
                      seq-local: [w331 _ _] -> [_ w399 _]
                      tunnel: w316 -> [w328 w409 w467]
                      tunnel: w315 -> [_ w428 _]
                      tunnel: w314 -> [_ w401 _]
                      tunnel: w313 -> [_ w423 _]
                      tunnel: w317 -> [w363 w400 _]
                      tunnel: w312 -> [_ _ _]
                      tunnel: w311 -> [_ _ _]
                      tunnel: w310 -> [w336 _ w478]
                      tunnel: w309 -> [_ _ w477]
                      tunnel: w308 -> [w321 w421 w462]
                      tunnel: w307 -> [_ _ w476]
                      tunnel: w306 -> [_ w402 _]
                      tunnel: w305 -> [_ _ w475]
                      tunnel: w304 -> [_ w408 _]
                      tunnel: w303 -> [_ _ w474]
                      tunnel: w302 -> [_ _ w472]
                      tunnel: w301 -> [_ w415 w471]
                      tunnel: w300 -> [_ _ w470]
                      tunnel: w299 -> [_ _ w465]
                      tunnel: w298 -> [w330 _ _]
                      frame #0 {
                        # "Val 33~56"
                        n198 = Select(t=2, s=w336, f=0) -> (s? t:f=w339:i32)
                        n199 = property on="108" class="Bool (strict)"("Disabled"=w339) -> ()  [unwired: 2 in, 2 out]
                        n200 = Build Array("33", "34", "35", "36", "37", "38", "39", "40", "41", "42", "43", "44", "45", "46", "47", "48", "49", "50", "51", "52", "53", "54", "55", "56") -> (w362:bool[])
                        n201 = Replace Array Subset(array=w363, new element=w362, index=u32 32) -> (w358:bool[])
                        n202 = Build Array("108", "109", "110", "111", "112") -> (w348:bool[])
                        n203 = Build Array("91", "92", "93", "94") -> (w360:bool[])
                        n204 = Build Array("28", FALSE ("Input Element"), "30", "31", "32") -> (w354:bool[])
                        n205 = Replace Array Subset(array=w358, new element="26", index=25 ("Index")) -> (w356:bool[])
                        n206 = Replace Array Subset(array=w356, new element=w354, index=u32 27) -> (w349:bool[])
                        n207 = Replace Array Subset(array=w349, new element=w360, index=u32 90 ("Start Index")) -> (w347:bool[])
                        n208 = Replace Array Subset(array=w347, new element=w348, index=u32 107) -> (w322:bool[])
                        n209 = Replace Array Subset(array=w322, new element="97", index=u32 96) -> (w332:bool[])
                        n210 = Compound Arithmetic op=AND("123", w321) -> (w319:bool)
                        n211 = case shown="True" w319 {
                          tunnel: "123" -> [w390 w392]
                          tunnel: [w390 w391] -> w320
                          frame False {
                          }
                          frame True {
                            n212 = Not(x=w392) -> (.not. x?=w391:bool)
                            n213 = local write "123"(w391) -> ()
                          }
                        }
                        n214 = Replace Array Subset(array=w332, new element=w320, index=122 ("Index")) -> (w331:bool[])
                        n215 = Index Array(array=w331, index=w330) -> (element=w329:bool)
                        n216 = Not Equal?(x=w329, y=w320) -> (x != y?=w327:bool)
                        n217 = Compound Arithmetic op=AND(w327, w328) -> (w326:bool)
                        n218 = case shown="True" w326 {
                          tunnel: w330 -> [_ w394]
                          tunnel: w320 -> [_ w393]
                          frame False {
                          }
                          frame True {
                            n219 = global read "DynaGlbs.vi" "Valves rcp"() -> (w396:bool[])
                            n220 = Replace Array Subset(array=w396, new element=w393, index=w394) -> (w395:bool[])
                            n221 = global write "DynaGlbs.vi" "Valves rcp"(w395) -> ()
                          }
                        }
                      }
                      frame #1 {
                        # "System Dependent"
                        # "Set Valve States"
                        n222 = Not Equal?(x=u8 10, y=w415) -> (x != y?=w417:bool)
                        n223 = Or(x=w421, y=w409) -> (x .or. y?=w422:bool)
                        n224 = global read "ScrnGlbs.vi" "DinSpec"() -> (w404:bool)
                        n225 = case shown="True" w404 {
                          tunnel: [w429 w436] -> w403
                          tunnel: w400 -> [w433 _]
                          tunnel: 103 -> [w432 _]
                          tunnel: TRUE -> [w431 _]
                          tunnel: u32 0 -> [w430 _]
                          tunnel: w408 -> [_ w434]
                          frame False {
                            n226 = Index Array(array=w433, index=w432) -> (element=w429:bool)
                            n227 = local write "104"(w429) -> ()
                            n228 = global write "DynaGlbs.vi" "N2 Timer"(w430) -> ()
                            n229 = global write "ScrnGlbs.vi" "DinSpec"(w431) -> ()
                          }
                          frame True {
                            n230 = call "EBARA_Timer.vi"("Time Intv"=w434) -> ("N2 Valve"=w435:bool)
                            n231 = case shown="True" w435 {
                              selector: w435 -> [w437 _]
                              tunnel: [w437 "104"] -> w436
                              frame False {
                                n232 = local write "104"(w437) -> ()
                              }
                              frame True {
                              }
                            }
                          }
                        }
                        n233 = global read "DynaGlbs.vi" "GV/Vac?"() -> (w414:bool)
                        n234 = And(x=w417, y=w414) -> (x .and. y?=w413:bool)
                        n235 = case shown="False" w413 {
                          tunnel: [w440 "103"] -> w418
                          tunnel: w400 -> [w441 _]
                          tunnel: w402 -> [w439 _]
                          frame False {
                            n236 = Index Array(array=w441, index=w439) -> (element=w440:bool)
                            n237 = local write "103"(w440) -> ()
                          }
                          frame True {
                          }
                        }
                        n238 = Not(x=w414) -> (.not. x?=w419:bool)
                        n239 = property on="Vac lock" class="Str"("Visible"=w419) -> ()  [unwired: 2 in, 2 out]
                        n240 = Build Array("101", "val102", w418, w403) -> (w411:bool[])
                        n241 = Replace Array Subset(array=w399, new element=w411, index=u32 100) -> (w410:bool[])
                        n242 = case shown="False" w422 {
                          tunnel: w410 -> [w457 w461]
                          tunnel: w428 -> [w456 w460]
                          tunnel: [w454 w461] -> w420
                          frame False {
                            n243 = local read "LL Door"() -> (w453:bool)
                            n244 = Not(x=w453) -> (.not. x?=w455:bool)
                            n245 = Replace Array Subset(array=w457, new element=w455, index=w456) -> (w454:bool[])
                          }
                          frame True {
                            n246 = Index Array(array=w461, index=w460) -> (element=w459:bool)
                            n247 = Not(x=w459) -> (.not. x?=w458:bool)
                            n248 = local write "LL Door"(w458) -> ()
                          }
                        }
                        n249 = Not Equal?(x=w400, y=w420) -> (x != y?=w427:bool[])
                        n250 = Build Array(1) -> (w425:i32[])
                        n251 = Or Array Elements(Boolean array=w427) -> (logical OR=w424:bool)
                        n252 = case shown="True" w424 {
                          selector: w424 -> [_ w447]
                          tunnel: w425 -> [_ w444]
                          tunnel: w401 -> [_ w446]
                          tunnel: w420 -> [_ w445]
                          tunnel: w423 -> [_ w443]
                          frame False {
                          }
                          frame True {
                            n253 = case shown="False" w443 {
                              tunnel: w447 -> [w451 _]
                              tunnel: w446 -> [w450 _]
                              tunnel: w445 -> [w449 w452]
                              tunnel: w444 -> [w448 _]
                              frame False {
                                n254 = call "DOut.vi"("Dout[]"=w449, "ch#s"=w448, "Single?"=w450, "all"=w451) -> ()  [unwired: 1 in, 2 out]
                              }
                              frame True {
                                n255 = global write "DynaGlbs.vi" "Valves"(w452) -> ()
                              }
                            }
                          }
                        }
                        "val102 2" <- "val102"
                      }
                      frame #2 {
                        n256 = In Range and Coerce(upper limit=w472, x=w471, lower limit=w470) -> (In Range?=w469:bool)  [unwired: 1 out]
                        n257 = global read "ScrnGlbs.vi" "GV Down"() -> (w463:bool)
                        n258 = Equal?(x=w463, y=w462) -> (x = y?=w464:bool)
                        n259 = Compound Arithmetic op=OR(w465, w464, w469, w467) -> (w468:bool)
                        n260 = case shown="False" w468 {
                          tunnel: w478 -> [w490 _]
                          tunnel: w477 -> [w489 _]
                          tunnel: w462 -> [w486 w533]
                          tunnel: w476 -> [w485 _]
                          tunnel: w475 -> [w483 _]
                          tunnel: w474 -> [w482 _]
                          tunnel: [w481 w533] -> w466
                          tunnel: [w480 w532] -> w473
                          tunnel: w463 -> [w479 w532]
                          frame False {
                            n261 = Not Equal?(x="GV Up", y=w486) -> (x != y?=w487:bool)
                            n262 = Not Equal?(x=w479, y="GV Down") -> (x != y?=w492:bool)
                            n263 = Or(x=w487, y=w492) -> (x .or. y?=w484:bool)
                            n264 = case shown="False" w490 {
                              tunnel: "GV Up" -> [w503 _]
                              tunnel: w487 -> [w502 _]
                              tunnel: w489 -> [w501 _]
                              tunnel: "GV Down" -> [w500 _]
                              tunnel: w485 -> [_ w520]
                              tunnel: w486 -> [w499 w525]
                              tunnel: w479 -> [w498 w524]
                              tunnel: w484 -> [w497 _]
                              tunnel: [w496 w523] -> w481
                              tunnel: [w495 w522] -> w480
                              tunnel: w483 -> [w494 w521]
                              tunnel: w482 -> [w493 _]
                              frame False {
                                n265 = case shown="True" w497 {
                                tunnel: w503 -> [_ w512]
                                tunnel: w500 -> [_ w511]
                                tunnel: w502 -> [_ w513]
                                tunnel: w501 -> [_ w510]
                                tunnel: [w505 w509] -> w496
                                tunnel: [w504 w508] -> w495
                                tunnel: w499 -> [w505 _]
                                tunnel: w498 -> [w504 _]
                                tunnel: w494 -> [_ w507]
                                tunnel: w493 -> [_ w506]
                                frame False {
                                }
                                frame True {
                                n266 = case shown="True" w513 {
                                tunnel: w512 -> [w516 w519]
                                tunnel: [w515 w519] -> w509
                                tunnel: w511 -> [w514 w518]
                                tunnel: [w514 w517] -> w508
                                frame False {
                                n267 = Not(x=w516) -> (.not. x?=w515:bool)
                                }
                                frame True {
                                n268 = Not(x=w518) -> (.not. x?=w517:bool)
                                }
                                }
                                n269 = call "Door_Rout.vi"("GV/LL"=w507, "MCP"=w506, "manual"=w510, "Open/Close"=w509) -> ()  [unwired: 2 in, 1 out]
                                }
                                }
                              }
                              frame True {
                                n270 = case shown="True" w525 {
                                selector: w525 -> [w527 w530]
                                tunnel: [w527 w531] -> w523
                                tunnel: [w526 w530] -> w522
                                tunnel: w524 -> [w526 _]
                                tunnel: w521 -> [_ w529]
                                tunnel: w520 -> [_ w528]
                                frame False {
                                }
                                frame True {
                                w531 = FALSE
                                n271 = call "Door_Rout.vi"("GV/LL"=w529, "MCP"=w528, "manual"=w530, "Open/Close"=w531) -> ()  [unwired: 2 in, 1 out]
                                }
                                }
                              }
                            }
                          }
                          frame True {
                          }
                        }
                        n272 = local write "GV Down"(w473) -> ()
                        n273 = local write "GV Up"(w466) -> ()
                      }
                    }
                  }
                }
              }
              frame True {
                # "System Dependent"
                n274 = Index Array(array=w534, index=w597) -> (element=w596:bool)
                n275 = Array Subset(array=w534, index=25, length=36) -> (w599:bool[])
                n276 = Not(x=w596) -> (.not. x?=w595:bool)
                n277 = Array To Cluster(array=w599) -> (cluster=w600:T11)
                n278 = local write "LL Door"(w595) -> ()
                n279 = Unbundle(w600) -> ("[0]"=w582:bool, "[2]"=w538:bool, "[4]"=w537:bool, "[5]"=w536:bool, "[6]"=w535:bool, "[7]"=w581:bool, "[8]"=w580:bool, "[9]"=w579:bool, "[10]"=w578:bool, "[11]"=w577:bool, "[12]"=w576:bool, "[13]"=w575:bool, "[14]"=w574:bool, "[15]"=w573:bool, "[16]"=w572:bool, "[17]"=w571:bool, "[18]"=w570:bool, "[19]"=w569:bool, "[20]"=w568:bool, "[21]"=w567:bool, "[22]"=w566:bool, "[23]"=w565:bool, "[24]"=w564:bool, "[25]"=w563:bool, "[26]"=w562:bool, "[27]"=w561:bool, "[28]"=w560:bool, "[29]"=w559:bool, "[30]"=w558:bool)  [unwired: 7 out]
                n280 = local write "52"(w562) -> ()
                n281 = local write "26"(w582) -> ()
                n282 = local write "42"(w572) -> ()
                n283 = local write "47"(w567) -> ()
                n284 = local write "37"(w577) -> ()
                n285 = local write "32"(w535) -> ()
                n286 = local write "28"(w538) -> ()
                n287 = local write "53"(w561) -> ()
                n288 = local write "33"(w581) -> ()
                n289 = local write "43"(w571) -> ()
                n290 = local write "48"(w566) -> ()
                n291 = local write "38"(w576) -> ()
                n292 = local write "30"(w537) -> ()
                n293 = local write "34"(w580) -> ()
                n294 = local write "44"(w570) -> ()
                n295 = local write "49"(w565) -> ()
                n296 = local write "39"(w575) -> ()
                n297 = local write "54"(w560) -> ()
                n298 = local write "31"(w536) -> ()
                n299 = local write "55"(w559) -> ()
                n300 = local write "35"(w579) -> ()
                n301 = local write "45"(w569) -> ()
                n302 = local write "50"(w564) -> ()
                n303 = local write "40"(w574) -> ()
                n304 = local write "51"(w563) -> ()
                n305 = local write "56"(w558) -> ()
                n306 = local write "36"(w578) -> ()
                n307 = local write "46"(w568) -> ()
                n308 = local write "41"(w573) -> ()
                n309 = Array Subset(array=w534, index=90, length=4) -> (w587:bool[])
                n310 = Index Array(array=w534, index=122) -> (element=w541:bool)
                n311 = Index Array(array=w534, index=96) -> (element=w544:bool)
                n312 = Array Subset(array=w534, index=100, length=4) -> (w590:bool[])
                n313 = Array Subset(array=w534, index=107, length=5) -> (w585:bool[])
                n314 = Array To Cluster(array=w587) -> (cluster=w586:T12)
                n315 = Array To Cluster(array=w590) -> (cluster=w540:T12)
                n316 = Array To Cluster(array=w585) -> (cluster=w546:T13)
                n317 = local write "123"(w541) -> ()
                n318 = local write "97"(w544) -> ()
                n319 = Unbundle(w540) -> ("[0]"=w539:bool, "[1]"=w557:bool, "[2]"=w556:bool, "[3]"=w555:bool)
                n320 = Unbundle(w586) -> ("[0]"=w550:bool, "[1]"=w549:bool, "[2]"=w548:bool, "[3]"=w547:bool)
                n321 = Unbundle(w546) -> ("[0]"=w545:bool, "[1]"=w554:bool, "[2]"=w553:bool, "[3]"=w552:bool, "[4]"=w551:bool)
                n322 = local write "108"(w545) -> ()
                n323 = local write "91"(w550) -> ()
                n324 = local write "101"(w539) -> ()
                n325 = local write "92"(w549) -> ()
                n326 = local write "109"(w554) -> ()
                n327 = local write "val102"(w557) -> ()
                n328 = local write "93"(w548) -> ()
                n329 = local write "110"(w553) -> ()
                n330 = global write "DynaGlbs.vi" "New Dout"(w598) -> ()
                n331 = local write "94"(w547) -> ()
                n332 = local write "103"(w556) -> ()
                n333 = local write "111"(w552) -> ()
                n334 = local write "104"(w555) -> ()
                n335 = local write "112"(w551) -> ()
              }
            }
          }
          frame #1 {
            n336 = global read "RcpGlbs.vi" "Total Layers"() -> (w612:u8)
            n337 = global read "DynaGlbs.vi" "New Aout"() -> (w615:bool)
            n338 = global read "DynaGlbs.vi" "AOUTS"() -> (w619:dbl[])
            n339 = Or(x=w617, y=w615) -> (x .or. y?=w616:bool)
            n340 = call "RampChg.vi"("Action"=enum16{"Init", "Read", "Set"}."Read") -> ("Ramp Chg"=w624:bool[])  [unwired: 2 in, 1 out]
            n341 = Greater?(x=w612, y=1) -> (0:w611:bool)
            n342 = case shown="True" w616 {
              tunnel: w625 -> [_ w720]
              tunnel: w626 -> [_ w723]
              tunnel: w619 -> [w640 w721]
              tunnel: w624 -> [_ w722]
              tunnel: w623 -> [w641 _]
              tunnel: w622 -> [w639 _]
              tunnel: w621 -> [w638 w717]
              tunnel: w617 -> [_ w718]
              tunnel: w620 -> [w637 _]
              tunnel: w614 -> [_ w716]
              tunnel: w611 -> [_ w715]
              tunnel: w610 -> [w636 _]
              tunnel: [w635 w714] -> w609
              tunnel: w608 -> [w634 _]
              tunnel: w607 -> [w633 _]
              tunnel: w606 -> [w632 _]
              tunnel: w605 -> [w631 _]
              tunnel: [w630 w713] -> w604
              tunnel: [w629 w712] -> w603
              tunnel: [w628 w711] -> w602
              tunnel: [w627 w710] -> w601
              frame False {
                n343 = case shown="True" w638 {
                  tunnel: w640 -> [_ w708]
                  tunnel: w641 -> [_ _]
                  tunnel: w639 -> [_ w679]
                  tunnel: w637 -> [_ _]
                  tunnel: w636 -> [w646 w707]
                  tunnel: [w646 w706] -> w635
                  tunnel: w634 -> [w645 w700]
                  tunnel: w633 -> [w644 w692]
                  tunnel: w632 -> [w643 w691]
                  tunnel: w631 -> [w642 w690]
                  tunnel: [w645 w675] -> w630
                  tunnel: [w644 w674] -> w629
                  tunnel: [w643 w673] -> w628
                  tunnel: [w642 w672] -> w627
                  frame False {
                  }
                  frame True {
                    w658 = 0.0
                    w669 = 0.0 ("Input Element")
                    # "System Dependent"
                    n344 = Build Array("Fout38", w658, w658, "Fout41") -> (w673:dbl[])
                    n345 = Build Array("Fout25", "Fout26", w669, w669, "Fout29", "Fout30") -> (w706:dbl[])
                    n346 = Build Array("Fout83", "Fout84", "Fout85", 0.0 ("Input Element"), "Fout87", "Fout88") -> (w675:dbl[])
                    n347 = Not Equal?(x=w691, y=w673) -> (x != y?=w693:bool[])
                    n348 = Not Equal?(x=w700, y=w675) -> (x != y?=w699:bool[])
                    n349 = Not Equal?(x=w707, y=w706) -> (x != y?=w703:bool[])
                    n350 = Or Array Elements(Boolean array=w693) -> (logical OR=w694:bool)
                    n351 = Or Array Elements(Boolean array=w699) -> (logical OR=w698:bool)
                    n352 = Or Array Elements(Boolean array=w703) -> (logical OR=w702:bool)
                    n353 = call "Manu_Aout_Change.vi"("Aout_changed?"=w702, "Length"=u8 6, "Start_Index"=u8 24, "Sub_Aout"=w706, "G_Aouts"=w708) -> ("Aout_out"=w701:dbl[])  [unwired: 1 in]
                    n354 = call "Manu_Aout_Change.vi"("Aout_changed?"=w698, "Length"=u8 6, "Start_Index"=u8 82, "Sub_Aout"=w675, "G_Aouts"=w701) -> ("Aout_out"=w695:dbl[])  [unwired: 1 in]
                    n355 = call "Manu_Aout_Change.vi"("Off_Line"=w679, "Aout_changed?"=w694, "Length"=u8 4, "Start_Index"=u8 37, "Sub_Aout"=w673, "G_Aouts"=w695) -> ("Aout_out"=w678:dbl[])
                    n356 = Build Array("Fout73", "Fout74", "Fout75", "Fout76") -> (w672:dbl[])
                    n357 = Build Array("Fout49", "Fout50", "Fout51", "Fout52", "Fout53", "Fout54", "Fout55") -> (w674:dbl[])
                    n358 = Not Equal?(x=w672, y=w690) -> (x != y?=w689:bool[])
                    n359 = Not Equal?(x=w674, y=w692) -> (x != y?=w683:bool[])
                    n360 = Or Array Elements(Boolean array=w689) -> (logical OR=w688:bool)
                    n361 = Or Array Elements(Boolean array=w683) -> (logical OR=w682:bool)
                    n362 = call "Manu_Aout_Change.vi"("Aout_changed?"=w682, "Length"=u8 7, "Start_Index"=u8 48, "Sub_Aout"=w674, "G_Aouts"=w678) -> ("Aout_out"=w677:dbl[])  [unwired: 1 in]
                    n363 = call "Manu_Aout_Change.vi"("Off_Line"=w679, "Aout_changed?"=w688, "Length"=u8 4, "Start_Index"=u8 72, "Sub_Aout"=w672, "G_Aouts"=w677) -> ("Aout_out"=w676:dbl[])
                    n364 = case shown="True" w679 {
                      tunnel: w676 -> [_ w709]
                      frame False {
                      }
                      frame True {
                        n365 = global write "DynaGlbs.vi" "AOUTS"(w709) -> ()
                      }
                    }
                  }
                }
              }
              frame True {
                n366 = Compound Arithmetic op=AND(w717, invert w718, w720, w715) -> (w719:bool)
                n367 = stacked-sequence {
                  tunnel: w719 -> [w802 _]
                  tunnel: w723 -> [w803 _]
                  tunnel: w722 -> [w801 _]
                  tunnel: w721 -> [w733 w831]
                  tunnel: w716 -> [_ w842]
                  tunnel: [_ w830] -> w714
                  tunnel: [_ w829] -> w713
                  tunnel: [_ w828] -> w712
                  tunnel: [_ w827] -> w711
                  tunnel: [_ w826] -> w710
                  frame #0 {
                    w794 = 24
                    w793 = 6
                    w787 = 7
                    w788 = 48
                    w775 = 4
                    w776 = 37
                    w781 = 6
                    w782 = 82
                    w800 = 72
                    w799 = 4
                    # "System Dependent"
                    n368 = Select(t=w801, s=w802, f=w803) -> (s? t:f=w732:bool[])
                    n369 = Array Subset(array=w733, index=w782, length=w781) -> (w780:dbl[])
                    n370 = Array Subset(array=w732, index=w782, length=w781) -> (w779:bool[])
                    n371 = Array Subset(array=w733, index=w794, length=w793) -> (w792:dbl[])
                    n372 = Array Subset(array=w732, index=w794, length=w793) -> (w791:bool[])
                    n373 = Array Subset(array=w733, index=w788, length=w787) -> (w786:dbl[])
                    n374 = Array Subset(array=w732, index=w788, length=w787) -> (w785:bool[])
                    n375 = Array Subset(array=w733, index=w776, length=w775) -> (w774:dbl[])
                    n376 = Array Subset(array=w732, index=w776, length=w775) -> (w772:bool[])
                    n377 = Array To Cluster(array=w780) -> (cluster=w777:T6)
                    n378 = Array To Cluster(array=w779) -> (cluster=w778:T14)
                    n379 = Array To Cluster(array=w792) -> (cluster=w789:T6)
                    n380 = Array To Cluster(array=w791) -> (cluster=w790:T14)
                    n381 = Array To Cluster(array=w786) -> (cluster=w783:T7)
                    n382 = Array To Cluster(array=w785) -> (cluster=w784:T15)
                    n383 = Array To Cluster(array=w772) -> (cluster=w771:T12)
                    n384 = Array To Cluster(array=w774) -> (cluster=w773:T9)
                    n385 = Unbundle(w789) -> ("[0]"=w769:dbl, "[1]"=w768:dbl, "[4]"=w767:dbl, "[5]"=w766:dbl)  [unwired: 2 out]
                    n386 = Unbundle(w790) -> ("[0]"=w765:bool, "[1]"=w764:bool, "[4]"=w763:bool, "[5]"=w762:bool)  [unwired: 2 out]
                    n387 = Unbundle(w783) -> ("[0]"=w761:dbl, "[1]"=w760:dbl, "[2]"=w759:dbl, "[3]"=w758:dbl, "[4]"=w757:dbl, "[5]"=w756:dbl, "[6]"=w755:dbl)
                    n388 = Unbundle(w784) -> ("[0]"=w754:bool, "[1]"=w753:bool, "[2]"=w752:bool, "[3]"=w751:bool, "[4]"=w750:bool, "[5]"=w749:bool, "[6]"=w748:bool)
                    n389 = Unbundle(w771) -> ("[0]"=w734:bool, "[3]"=w735:bool)  [unwired: 2 out]
                    n390 = Unbundle(w777) -> ("[0]"=w747:dbl, "[1]"=w746:dbl, "[2]"=w745:dbl, "[4]"=w744:dbl, "[5]"=w743:dbl)  [unwired: 1 out]
                    n391 = Unbundle(w778) -> ("[0]"=w742:bool, "[1]"=w741:bool, "[2]"=w740:bool, "[4]"=w739:bool, "[5]"=w738:bool)  [unwired: 1 out]
                    n392 = Unbundle(w773) -> ("[0]"=w737:dbl, "[3]"=w736:dbl)  [unwired: 2 out]
                    n393 = case shown="True" w765 {
                      tunnel: w769 -> [_ w825]
                      frame False {
                      }
                      frame True {
                        n394 = local write "Fout25"(w825) -> ()
                      }
                    }
                    n395 = global read "RobotGlbs.vi" "LL Req"() -> (w770:bool)
                    n396 = case shown="True" w754 {
                      tunnel: w761 -> [_ w821]
                      frame False {
                      }
                      frame True {
                        n397 = local write "Fout49"(w821) -> ()
                      }
                    }
                    n398 = case shown="True" w742 {
                      tunnel: w747 -> [_ w815]
                      frame False {
                      }
                      frame True {
                        n399 = local write "Fout83"(w815) -> ()
                      }
                    }
                    n400 = Select(t=w770, s=w770, f=w735) -> ()  [unwired: 1 out]
                    n401 = case shown="True" w734 {
                      tunnel: w737 -> [_ w805]
                      frame False {
                      }
                      frame True {
                        n402 = local write "Fout38"(w805) -> ()
                      }
                    }
                    n403 = case shown="True" w764 {
                      tunnel: w768 -> [_ w824]
                      frame False {
                      }
                      frame True {
                        n404 = local write "Fout26"(w824) -> ()
                      }
                    }
                    n405 = case shown="True" w753 {
                      tunnel: w760 -> [_ w820]
                      frame False {
                      }
                      frame True {
                        n406 = local write "Fout50"(w820) -> ()
                      }
                    }
                    n407 = case shown="True" w741 {
                      tunnel: w746 -> [_ w814]
                      frame False {
                      }
                      frame True {
                        n408 = local write "Fout84"(w814) -> ()
                      }
                    }
                    n409 = case shown="True" w735 {
                      tunnel: w736 -> [_ w804]
                      frame False {
                      }
                      frame True {
                        n410 = local write "Fout41"(w804) -> ()
                      }
                    }
                    n411 = case shown="True" w763 {
                      tunnel: w767 -> [_ w823]
                      frame False {
                      }
                      frame True {
                        n412 = local write "Fout29"(w823) -> ()
                      }
                    }
                    n413 = case shown="True" w740 {
                      tunnel: w745 -> [_ w810]
                      frame False {
                      }
                      frame True {
                        n414 = local write "Fout85"(w810) -> ()
                      }
                    }
                    n415 = case shown="True" w752 {
                      tunnel: w759 -> [_ w819]
                      frame False {
                      }
                      frame True {
                        n416 = local write "Fout51"(w819) -> ()
                      }
                    }
                    n417 = case shown="True" w762 {
                      tunnel: w766 -> [_ w822]
                      frame False {
                      }
                      frame True {
                        n418 = local write "Fout30"(w822) -> ()
                      }
                    }
                    n419 = case shown="True" w739 {
                      tunnel: w744 -> [_ w812]
                      frame False {
                      }
                      frame True {
                        n420 = local write "Fout87"(w812) -> ()
                      }
                    }
                    n421 = case shown="True" w751 {
                      tunnel: w758 -> [_ w818]
                      frame False {
                      }
                      frame True {
                        n422 = local write "Fout52"(w818) -> ()
                      }
                    }
                    n423 = case shown="True" w738 {
                      tunnel: w743 -> [_ w811]
                      frame False {
                      }
                      frame True {
                        n424 = local write "Fout88"(w811) -> ()
                      }
                    }
                    n425 = Array Subset(array=w733, index=w800, length=w799) -> (w798:dbl[])
                    n426 = Array Subset(array=w732, index=w800, length=w799) -> (w797:bool[])
                    n427 = case shown="True" w750 {
                      tunnel: w757 -> [_ w817]
                      frame False {
                      }
                      frame True {
                        n428 = local write "Fout53"(w817) -> ()
                      }
                    }
                    n429 = Array To Cluster(array=w797) -> (cluster=w796:T12)
                    n430 = Array To Cluster(array=w798) -> (cluster=w795:T9)
                    n431 = Unbundle(w796) -> ("[0]"=w727:bool, "[1]"=w726:bool, "[2]"=w725:bool, "[3]"=w724:bool)
                    n432 = Unbundle(w795) -> ("[0]"=w731:dbl, "[1]"=w730:dbl, "[2]"=w729:dbl, "[3]"=w728:dbl)
                    n433 = case shown="True" w749 {
                      tunnel: w756 -> [_ w816]
                      frame False {
                      }
                      frame True {
                        n434 = local write "Fout54"(w816) -> ()
                      }
                    }
                    n435 = case shown="True" w727 {
                      tunnel: w731 -> [_ w809]
                      frame False {
                      }
                      frame True {
                        n436 = local write "Fout73"(w809) -> ()
                      }
                    }
                    n437 = case shown="True" w748 {
                      tunnel: w755 -> [_ w813]
                      frame False {
                      }
                      frame True {
                        n438 = local write "Fout55"(w813) -> ()
                      }
                    }
                    n439 = case shown="True" w726 {
                      tunnel: w730 -> [_ w808]
                      frame False {
                      }
                      frame True {
                        n440 = local write "Fout74"(w808) -> ()
                      }
                    }
                    n441 = case shown="True" w725 {
                      tunnel: w729 -> [_ w807]
                      frame False {
                      }
                      frame True {
                        n442 = local write "Fout75"(w807) -> ()
                      }
                    }
                    n443 = case shown="True" w724 {
                      tunnel: w728 -> [_ w806]
                      frame False {
                      }
                      frame True {
                        n444 = local write "Fout76"(w806) -> ()
                      }
                    }
                  }
                  frame #1 {
                    # "System Dependent"
                    n445 = Array Subset(array=w831, index=24, length=6) -> (w830:dbl[])
                    n446 = Array Subset(array=w831, index=82, length=6) -> (w829:dbl[])
                    n447 = Array Subset(array=w831, index=48, length=7) -> (w828:dbl[])
                    n448 = Array Subset(array=w831, index=37, length=4) -> (w827:dbl[])
                    n449 = Array Subset(array=w831, index=72 ("Array Index"), length=4 ("Array Length")) -> (w826:dbl[])
                    n450 = global read "ScrnGlbs.vi" "temp done"() -> (w845:bool)
                    n451 = Not Or(1:w845, 2:w842) -> (0:w844:bool)
                    n452 = case shown="False" w844 {
                      selector: w844 -> [w846 w847]
                      tunnel: [w846 w847] -> w843
                      frame False {
                        n453 = global write "DynaGlbs.vi" "New Aout"(w846) -> ()
                        n454 = global write "ScrnGlbs.vi" "temp done"(w846) -> ()
                      }
                      frame True {
                      }
                    }
                    n455 = global write "ScrnGlbs.vi" "Scrn done"(w843) -> ()
                  }
                }
              }
            }
          }
        }
      }
    }
    n456 = global read "ScrnGlbs.vi" "exit"() -> (w180:bool)
    n457 = call "GaNLite_Flag.vi"("Selector"=enum16{"Start", "Check", "Stop"}."Check") -> ("Running"=w166:bool)  [unwired: 1 in]
    n458 = property on="PP Rout" class="Str"("Blinking"=w166) -> ()  [unwired: 2 in, 2 out]
    n459 = property on="PP Rout" class="Str"("Visible"=w166) -> ()  [unwired: 2 in, 2 out]
  }
